vi "VapIn.vi"(11 "Abs. Pressure\nVoltage [V]":dbl) -> (3 "Absolute Pressure [kPa]":dbl)   [LabVIEW 2017]
uses:
  <vilib>/express/express arith-compare/Formula/XNode/ExpressFormulaBlockNode.xnode
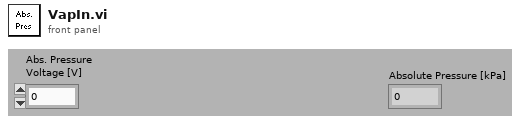
[diagram p1: front panel]
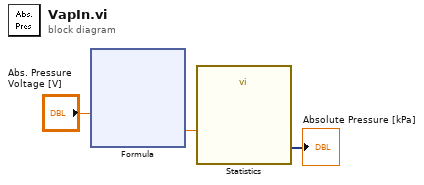
[diagram p0: block diagram]
diagram:
  n1 = xnode "Formula"("V"="Abs. Pressure\nVoltage [V]") -> ("Result"=w3:dbl)  [unwired: 1 in, 1 out]
  n2 = call "Statistics"("Signals"=w3) -> ("Arithmetic Mean"=→"Absolute Pressure [kPa]":dynamicdata)  [unwired: 25 in, 1 out]
